vi "18.6 Color Segmentation.vi"() -> ()   [LabVIEW 2017]
doc: "Demonstrates how to use the IMAQ Color Segmentation function to produce a segmented greyscale image where each color, defined in a color classifier file, has a unique greyscale value in the segmented image."
uses:
  <vilib>/vision/NI_Vision_Development_Module.lvlib
panel:
  out "Color Image":T1(plugin-control)
  out "Segmented Image":T1(plugin-control)
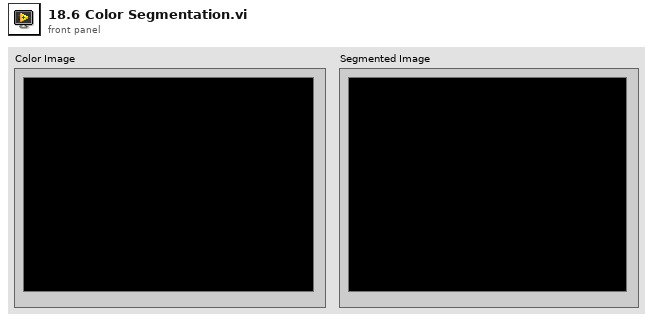
[diagram p1: front panel]
types:
  T1 = typedef "IMAQ Image.ctl" = refnum<image>
  T2 = typedef "Image Type" = u32
  T3 = cluster{"Window Size":cluster{"X":u32, "Y":u32}, "Step Size":u32, "Min Particle Area":u32, "Max Particle Area":u32, "Refine Segmentation?":bool}
  T4 = typedef "IMAQ Classifier Session.ctl" = refnum<k1>
  T5 = typedef "ROI Descriptor" = cluster{"Global Rectangle":i32[], "Contours":cluster{"ID":enum32{"External", "Internal"}, "Type":u32, "Coordinates":i32[]}[]}
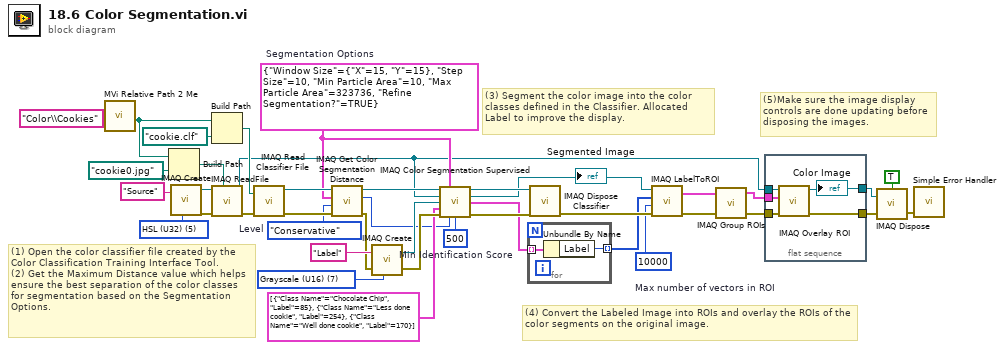
[diagram p0: block diagram]
diagram:
  w24 = 500  # Min Identification Score
  w27 = enum32{"Conservative", "Aggressive"}."Conservative"  # Level
  w35 = T2 7 items=["Grayscale (U8)", "Grayscale (I16)", "Grayscale (SGL)", "Complex (CSG)", "RGB (U32)", "HSL (U32)", "RGB (U64)", "Grayscale (U16)"] ("Image Type")
  w37 = T2 5 items=["Grayscale (U8)", "Grayscale (I16)", "Grayscale (SGL)", "Complex (CSG)", "RGB (U32)", "HSL (U32)", "RGB (U64)", "Grayscale (U16)"] ("Image Type")
  w18 = 10000  # Max number of vectors in ROI
  w26 = T3 {"Window Size"={"X"=15, "Y"=15}, "Step Size"=10, "Min Particle Area"=10, "Max Particle Area"=323736, "Refine Segmentation?"=TRUE}  # Segmentation Options
  # "(5)Make sure the image display controls are done updating before disposing the images."
  # "(4) Convert the Labeled Image into ROIs and overlay the ROIs of the color segments on the original image."
  # "(3) Segment the color image into the color classes defined in the Classifier. Allocated Label to improve the display."
  # "(1) Open the color classifier file created by the Color Classification Training Interface Tool. \n(2) Get the Maximum Distance value which helps ensure the best separation of the color classes for segmentation based on the Segmentation Options."
  n1 = call "MVi Relative Path 2 Me.vi"("Relative Path"="Color\\Cookies") -> ("Appended Dir"=w12:path)  [unwired: 5 in, 1 out]
  n2 = Build Path(base path=w12, name or relative path=path "cookie0.jpg") -> (appended path=w31:path)
  n3 = call "IMAQ Create"("Image Name"="Source", "Image Type"=w37) -> ("New Image"=w34:T1, "error out"=w33:errorcluster)  [unwired: 2 in, 1 out]
  n4 = Build Path(base path=w12, name or relative path=path "cookie.clf") -> (appended path=w38:path)
  n5 = call "IMAQ ReadFile"("File Path"=w31, "error in (no error)"=w33, "Image"=w34) -> ("error out"=w30:errorcluster, "Image Out"=w5:T1)  [unwired: 4 in, 3 out]
  n6 = call "IMAQ Read Classifier File"("File Path"=w38, "error in (no error)"=w30) -> ("error out"=w28:errorcluster, "Classifier Session"=w29:T4)  [unwired: 2 in, 6 out]
  n7 = call "IMAQ Get Color Segmentation Distance"("error in (no error)"=w28, "Level"=w27, "Segmentation Options"=w26, "Color Classifier Session"=w29) -> ("error out"=w11:errorcluster, "Maximum Distance"=w4:i32, "Color Classifier Session (dup)"=w16:T4)  [unwired: 5 in]
  n8 = call "IMAQ Create"("Image Name"="Label", "Image Type"=w35, "error in (no error)"=w11) -> ("New Image"=w25:T1, "error out"=w10:errorcluster)  [unwired: 1 in, 1 out]
  n9 = call "IMAQ Color Segmentation Supervised"("Color Classifier Session"=w16, "Segmentation Options"=w26, "Image"=w5, "Label Image"=w25, "Labels In"=cluster{"Class Name":string, "Label":u32}[] [{"Class Name"="Chocolate Chip", "Label"=85}, {"Class Name"="Less done cookie", "Label"=254}, {"Class Name"="Well done cookie", "Label"=170}] ("Labels"), "error in (no error)"=w10, "Maximum Distance"=w4, "Min Identification Score"=w24) -> ("Color Classifier Session (dup)"=w22:T4, "Label Image Out"=w1:T1, "Labels Out"=w20:cluster{"Class Name":string, "Label":u32}[], "error out"=w23:errorcluster)  [unwired: 1 in, 3 out]
  "Segmented Image" <- w1
  n10 = for {
    tunnel: w20 -> [w42] mode=indexing
    tunnel: [w41] -> w19 mode=indexing
    n11 = Unbundle By Name(w42) -> ("Label"=w41:u32)
  }
  n12 = call "IMAQ Dispose Classifier"("error in (no error)"=w23, "Classifier Session"=w22) -> ("error out"=w21:errorcluster)  [unwired: 9 out]
  n13 = call "IMAQ LabelToROI"("error in (no error)"=w21, "Max number of vectors in ROI"=w18, "Labels In"=w19, "Image"=w1) -> ("error out"=w6:errorcluster, "ROIs"=w14:T5[])  [unwired: 1 in, 5 out]
  n14 = call "IMAQ Group ROIs"("error in (no error)"=w6, "ROI Descriptors"=w14) -> ("error out"=w15:errorcluster, "ROI Descriptor out"=w17:T5)  [unwired: 2 in]
  n15 = flat-sequence {
    tunnel: w17 -> [w47]
    tunnel: w15 -> [w46]
    tunnel: w5 -> [w45]
    tunnel: [w44] -> w3
    tunnel: [w43] -> w2
    frame #0 {
      n16 = call "IMAQ Overlay ROI"("error in (no error)"=w46, "ROI Descriptor"=w47, "Image"=w45) -> ("error out"=w43:errorcluster, "Image Out"=w44:T1)  [unwired: 7 in]
      "Color Image" <- w44
    }
  }
  n17 = call "IMAQ Dispose"("All Images? (No)"=TRUE, "Image"=w3, "error in (no error)"=w2) -> ("error out"=w9:errorcluster)  [unwired: 3 out]
  n18 = call <vilib>:"Simple Error Handler.vi"("error in (no error)"=w9) -> ()  [unwired: 4 in, 5 out]
